vi "expandArray.vi"(11 "Array":dbl[][](array[numeric])) -> ()   [LabVIEW 2016]
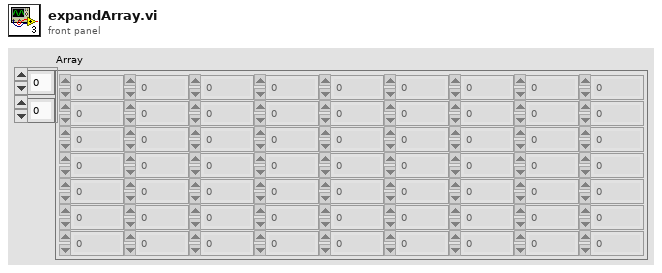
[diagram p1: front panel]
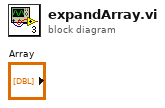
[diagram p0: block diagram]
diagram:
